vi "KE622x -- Get Math Mode Params.vi"(0 "Resource In":refnum<visa-resource-name>, 1 "Check For SCPI Errors? (T)":bool=TRUE, 11 "error in (no error)":errorcluster) -> (4 "Resource Out (dupl)":refnum<visa-resource-name>, 8 "Math Mode Params":T1={"Math Enabled?"=FALSE, "Math Mode"=enum."mX + b", "Slope (m)"=1.0, "Intercept (b)"=0.0} {"Intercept (b)" min=-9.99999e+20 max=9.99999e+20 format="%.5e"; "Slope (m)" min=-9.99999e+20 max=9.99999e+20 format="%.5e"}, 15 "error out":errorcluster)   [LabVIEW 2019, in "Keithley 622x.lvlib"]
doc: "Returns the math mode parameters for measurements returned from the 2182/2182A nano-voltmeter and also whether or not math mode is enabled."
uses:
  Keithley 622x.lvlib
  Typedefs/KE622x -- Math Mode Params.ctl
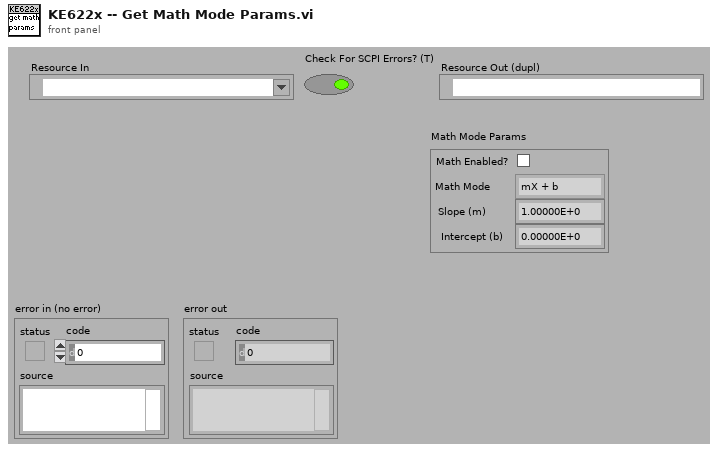
[diagram p1: front panel]
types:
  T1 = typedef "Keithley 622x.lvlib/KE622x -- Math Mode Params.ctl" = cluster{"Math Enabled?":bool, "Math Mode":enum16{"None", "mX + b", "m/X + b"}, "Slope (m)":dbl, "Intercept (b)":dbl}
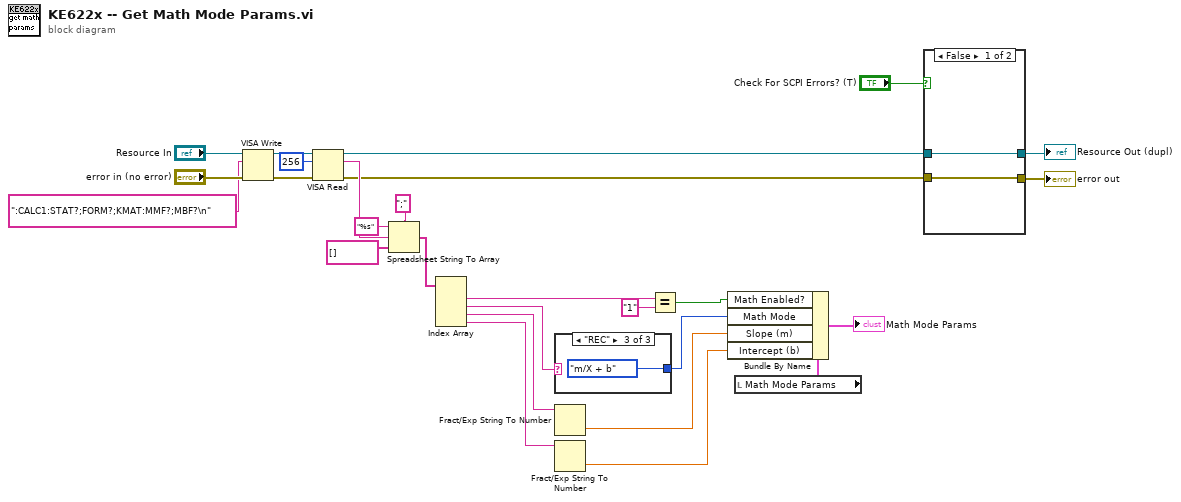
[diagram p0: block diagram]
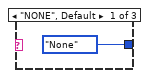
[diagram p2: hidden frame]
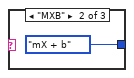
[diagram p3: hidden frame]
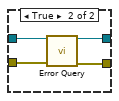
[diagram p4: hidden frame]
diagram:
  n1 = VISA Write(VISA resource name="Resource In", write buffer=":CALC1:STAT?;FORM?;KMAT:MMF?;MBF?\n" ("format string"), error in (no error)="error in (no error)") -> (VISA resource name out=w21:refnum<visa-resource-name>, error out=w20:errorcluster)  [unwired: 1 out]
  n2 = VISA Read(VISA resource name=w21, byte count=u32 256, error in (no error)=w20) -> (VISA resource name out=w18:refnum<visa-resource-name>, read buffer=w17:string, error out=w1:errorcluster)  [unwired: 1 out]
  n3 = Spreadsheet String To Array(delimiter (Tab)=";", format string="%s", spreadsheet string=w17, array type (2D Dbl)=string[] []) -> (array=w13:string[])
  n4 = Index Array(array=w13) -> (element #1=w12:string, element #2=w7:string, element #3=w6:string, element #4=w5:string)  [unwired: 4 in]
  n5 = case shown="\"REC\"" w7 {
    tunnel: [enum16{"None", "mX + b", "m/X + b"}."None" ("Math Mode") enum16{"None", "mX + b", "m/X + b"}."mX + b" ("Math Mode") enum16{"None", "mX + b", "m/X + b"}."m/X + b" ("Math Mode")] -> w4
    frame "NONE", Default {
    }
    frame "MXB" {
    }
    frame "REC" {
    }
  }
  n6 = Fract/Exp String To Number(string=w6) -> (number=w3:dbl)  [unwired: 3 in, 1 out]
  n7 = Fract/Exp String To Number(string=w5) -> (number=w2:dbl)  [unwired: 3 in, 1 out]
  n8 = Equal?(x=w12, y="1") -> (x = y?=w9:bool)
  n9 = local read "Math Mode Params"() -> (w10:T1)
  n10 = Bundle By Name(cluster=w10, "Math Enabled?"=w9, "Math Mode"=w4, "Slope (m)"=w3, "Intercept (b)"=w2) -> (→"Math Mode Params":T1)
  n11 = case shown="False" "Check For SCPI Errors? (T)" {
    tunnel: w18 -> [w32 w36]
    tunnel: w1 -> [w31 w35]
    tunnel: [w31 w34] -> w23
    tunnel: [w32 w33] -> w24
    frame False {
    }
    frame True {
      n12 = call "Error Query.vi"("VISA Resource In"=w36, "error in (no error)"=w35) -> ("VISA Resource Out (dupl)"=w33:refnum<visa-resource-name>, "error out"=w34:errorcluster)  [unwired: 10 in, 2 out]
    }
  }
  "Resource Out (dupl)" <- w24
  "error out" <- w23
